vi "XY Plot Commands.vi"(1 "X,Y Log":i32[](array[numeric])=[1, 0], 3 "input string":string="Display 'y_#wave#' vs 'x_#wave#'\nAppendToGraph 'y_#wave#' vs 'x_#wave#'\nLabel bottom \"#labelX#\"\nLabel left \"#labelY#\"\nModifyGraph rgb('y_#wave#')=(#r#,#g#,#b#)\n\\\\s('y_#wave#') #label#\nModifyGraph mirror=1\nModifyGraph width=216\nModifyGraph height={Aspect,0.6}\nModifyGraph Log(bottom)=#bottomlog#\nModifyGraph Log(left)=#leftlog#", 4 "Plot labels":string[](array[string])=["SR810 cables", "SR810 cables + 1&2", "detector", "cables", "cables + 1&2", "cables + 2&3", "cables + 3&4"], 5 "X,Y Labels":string[](array[string])=["frequency (Hz)", "V\\Brms\\M (V)"], 6 "wavenames":string[](array[string])=["Sum.000003SR810cables", "Sum.000003SR810cables + 1&2", "Sum.000003detector", "Sum.000003cables", "Sum.000003cables+ 1&2", "Sum.000003cables+ 2&3", "Sum.000003cables+ 3&4"]) -> (0 "result string":string="Display 'y_Sum.000003SR810cables' vs 'x_Sum.000003SR810cables'\nAppendToGraph 'y_Sum.000003SR810cables + 1&2' vs 'x_Sum.000003SR810cables + 1&2'\nAppendToGraph 'y_Sum.000003detector' vs 'x_Sum.000003detector'\nAppendToGraph 'y_Sum.000003cables' vs 'x_Sum.000003cables'\nAppendToGraph 'y_Sum.000003cables+ 1&2' vs 'x_Sum.000003cables+ 1&2'\nAppendToGraph 'y_Sum.000003cables+ 2&3' vs 'x_Sum.000003cables+ 2&3'\nAppendToGraph 'y_Sum.000003cables+ 3&4' vs 'x_Sum.000003cables+ 3&4'\nLabel bottom \"frequency (Hz)\"\nLabel left \"V\\Brms\\M (V)\"\nModifyGraph rgb('y_Sum.000003SR810cables')=(65280,0,0)\nModifyGraph rgb('y_Sum.000003SR810cables + 1&2')=(65280,50688,0)\nModifyGraph rgb('y_Sum.000003detector')=(29696,65280,0)\nModifyGraph rgb('y_Sum.000003cables')=(0,65280,20992)\nModifyGraph rgb('y_Sum.000003cables+ 1&2')=(0,60928,65280)\nModifyGraph rgb('y_Sum.000003cables+ 2&3')=(0,10240,65280)\nModifyGraph rgb('y_Sum.000003cables+ 3&4')=(40448,0,65280)\nLegend/C/N=text0/J \"\\\\s('y_Sum.000003SR810cables') SR810 cables\\r\\\\s('y_Sum.000003SR810cables + 1&2') SR810 cables + 1&2\\r\\\\s('y_Sum.000003detector') detector\\r\\\\s('y_Sum.000003cables') cables\\r\\\\s('y_Sum.000003cables+ 1&2') cables + 1&2\\r\\\\s('y_Sum.000003cables+ 2&3') cables + 2&3\\r\\\\s('y_Sum.000003cables+ 3&4') cables + 3&4\"\nModifyGraph mirror=1\nModifyGraph width=216\nModifyGraph height={Aspect,0.6}\n\n\n")   [LabVIEW 2016, in "LVtoITX.lvclass"]
uses:
  LVtoITX.lvclass
  <userlib>/LevyLab/Graph Utilities/graph_utilities.lvclass
panel:
  # "Legend/C/N=text0/J \"\\\\s('y_test.000011Plot9') Plot 9\\r\\\\s('y_test.000011Plot8') Plot 8\""
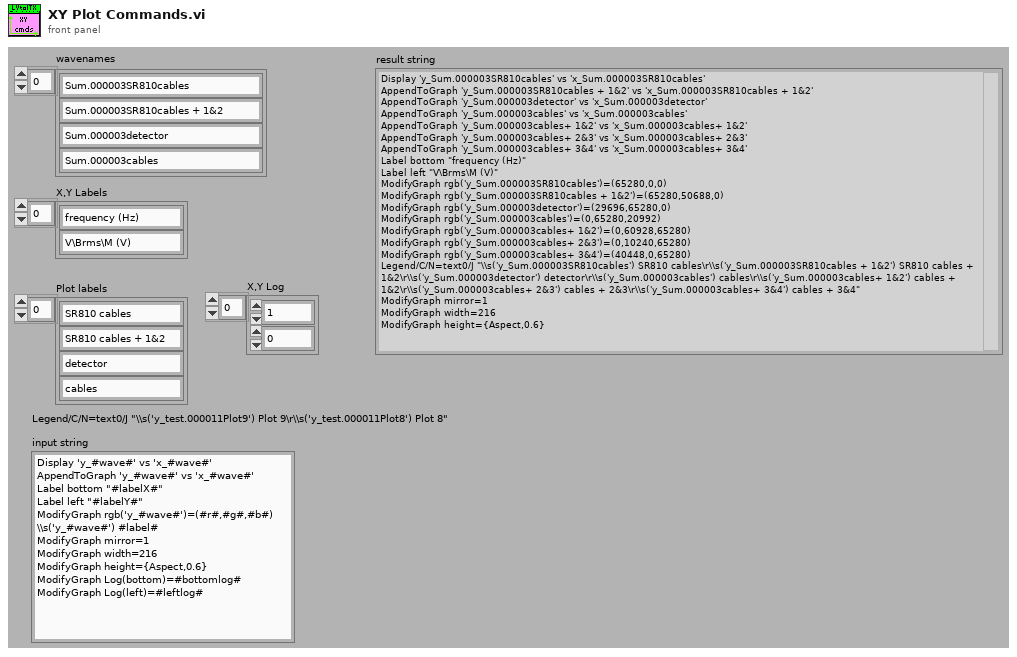
[diagram p1: front panel]
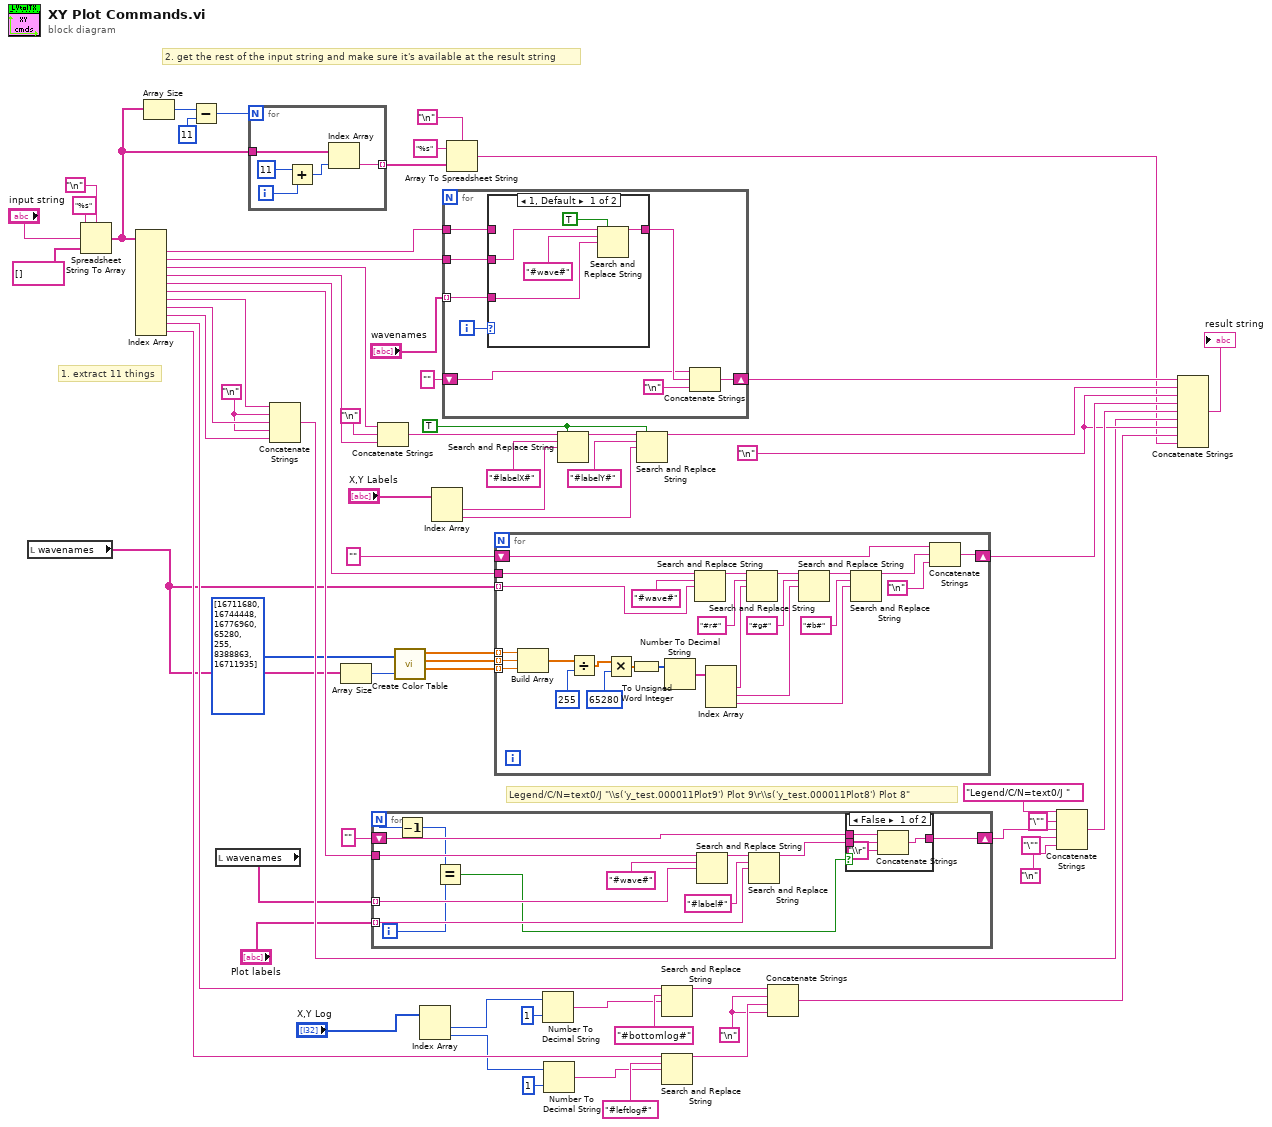
[diagram p0: block diagram]
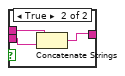
[diagram p2: hidden frame]
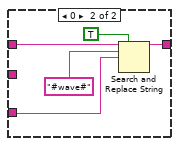
[diagram p3: hidden frame]
diagram:
  w25 = "\n"
  w34 = "\n"
  w33 = "\n"
  w55 = TRUE ("replace all? (F)")
  # "2. get the rest of the input string and make sure it's available at the result string"
  # "1. extract 11 things"
  # "Legend/C/N=text0/J \"\\\\s('y_test.000011Plot9') Plot 9\\r\\\\s('y_test.000011Plot8') Plot 8\""
  n1 = local read "wavenames"() -> (w1:string[])
  n2 = Spreadsheet String To Array(delimiter (Tab)="\n", format string="%s", spreadsheet string="input string", array type (2D Dbl)=string[] []) -> (array=w11:string[])
  n3 = Index Array(array=w11) -> (element #1=w63:string, element #2=w62:string, element #3=w47:string, element #4=w48:string, element #5=w49:string, element #6=w45:string, element #7=w44:string, element #8=w43:string, element #9=w35:string, element #10=w23:string, element #11=w22:string)  [unwired: 11 in]
  n4 = Array Size(array=w11) -> (size(s)=w14:i32)
  n5 = Subtract(x=w14, y=11 ("x")) -> (x-y=w12:i32)
  n6 = local read "wavenames"() -> (w29:string[])
  n7 = for {
    N: w12 -> [_]
    tunnel: w11 -> [w72]
    tunnel: [w71] -> w10 mode=indexing
    i -> [w74]
    n8 = Add(x=11, y=w74) -> (x+y=w75:i32)
    n9 = Index Array(array=w72, index=w75) -> (element=w71:string)
  }
  n10 = Concatenate Strings(w44, w34, w43, w34, w35) -> (w32:string)
  n11 = Array Size(array=w1) -> (size(s)=w6:i32)
  n12 = for {
    N -> [w79]
    shift-right: [w80] -> w38
    shift-left: "" -> [w87]
    tunnel: "Plot labels" -> [w81] mode=indexing
    tunnel: w45 -> [w84]
    tunnel: w29 -> [w83] mode=indexing
    i -> [w77]
    n13 = Decrement(x=w79) -> (x-1=w78:i32)
    n14 = Equal?(x=w78, y=w77) -> (x = y?=w76:bool)
    n15 = Search and Replace String(input string=w84, search string="#wave#", replace string=w83) -> (result string=w88:string)  [unwired: 1 in, 7 out]
    n16 = Search and Replace String(input string=w88, search string="#label#", replace string=w81) -> (result string=w82:string)  [unwired: 1 in, 7 out]
    n17 = case shown="False" w76 {
      tunnel: w87 -> [w92 w94]
      tunnel: w82 -> [w91 w93]
      tunnel: [w90 w95] -> w80
      frame False {
        n18 = Concatenate Strings(w92, w91, "\\r" ("string")) -> (w90:string)
      }
      frame True {
        n19 = Concatenate Strings(w94, w93) -> (w95:string)
      }
    }
  }
  n20 = Concatenate Strings(w47, "\n", w48) -> (w60:string)
  n21 = call <userlib>:"Create Color Table.vi"("Colors []"=u32[] [16711680, 16744448, 16776960, 65280, 255, 8388863, 16711935], "Size (256)"=w6) -> ("R []"=w5:dbl[], "G []"=w4:dbl[], "B []"=w3:dbl[])  [unwired: 1 out]
  n22 = Index Array(array="X,Y Log") -> (element #1=w16:i32, element #2=w15:i32)  [unwired: 2 in]
  n23 = Index Array(array="X,Y Labels") -> (element #1=w51:string, element #2=w50:string)  [unwired: 2 in]
  n24 = for {
    tunnel: "wavenames" -> [w101] mode=indexing
    tunnel: w63 -> [w103]
    tunnel: w62 -> [w102]
    shift-right: [w99] -> w67
    shift-left: "" -> [w96]
    i -> [w100]
    n25 = case shown="1, Default" w100 {
      tunnel: w103 -> [_ w111]
      tunnel: w102 -> [w106 _]
      tunnel: w101 -> [w107 w112]
      tunnel: [w105 w110] -> w98
      frame 1, Default {
        n26 = Search and Replace String(replace all?=TRUE ("replace all? (F)"), input string=w106, search string="#wave#", replace string=w107) -> (result string=w105:string)  [unwired: 1 in, 6 out]
      }
      frame 0 {
        n27 = Search and Replace String(replace all?=TRUE ("replace all? (F)"), input string=w111, search string="#wave#", replace string=w112) -> (result string=w110:string)  [unwired: 1 in, 6 out]
      }
    }
    n28 = Concatenate Strings(w96, w98, "\n") -> (w99:string)
  }
  n29 = Array To Spreadsheet String(delimiter (Tab)="\n", array=w10, 3:"%s" ("format string")) -> (spreadsheet string=w7:string)
  n30 = for {
    tunnel: w49 -> [w133]
    tunnel: w1 -> [w118] mode=indexing
    shift-right: [w130] -> w53
    shift-left: "" -> [w129]
    tunnel: w5 -> [w116] mode=indexing
    tunnel: w4 -> [w115] mode=indexing
    tunnel: w3 -> [w114] mode=indexing
    n31 = Build Array(w116, w115, w114) -> (w117:dbl[])
    n32 = Divide(x=w117, y=255) -> (x/y=w136:dbl[])
    n33 = Multiply(x=w136, y=65280) -> (x*y=w137:dbl[])
    n34 = To Unsigned Word Integer(number=w137) -> (unsigned 16bit integer=w135:u16[])
    n35 = Number To Decimal String(number=w135) -> (decimal integer string=w123:string[])  [unwired: 1 out]
    n36 = Search and Replace String(input string=w133, search string="#wave#", replace string=w118) -> (result string=w134:string)  [unwired: 1 in, 7 out]
    n37 = Index Array(array=w123) -> (element #1=w122:string, element #2=w121:string, element #3=w120:string)  [unwired: 3 in]
    n38 = Search and Replace String(input string=w134, search string="#r#", replace string=w122) -> (result string=w132:string)  [unwired: 1 in, 7 out]
    n39 = Search and Replace String(input string=w132, search string="#g#", replace string=w121) -> (result string=w131:string)  [unwired: 1 in, 7 out]
    n40 = Search and Replace String(input string=w131, search string="#b#", replace string=w120) -> (result string=w127:string)  [unwired: 1 in, 7 out]
    n41 = Concatenate Strings(w129, w127, "\n") -> (w130:string)
  }
  n42 = Number To Decimal String(number=w16, width (-)=i16 1) -> (decimal integer string=w18:string)
  n43 = Number To Decimal String(number=w15, width (-)=i16 1) -> (decimal integer string=w19:string)
  n44 = Search and Replace String(replace all?=w55, input string=w60, search string="#labelX#", replace string=w51) -> (result string=w58:string)  [unwired: 1 in, 6 out]
  n45 = Search and Replace String(replace all?=w55, input string=w58, search string="#labelY#", replace string=w50) -> (result string=w46:string)  [unwired: 1 in, 6 out]
  n46 = Search and Replace String(input string=w23, search string="#bottomlog#", replace string=w18) -> (result string=w27:string)  [unwired: 1 in, 7 out]
  n47 = Search and Replace String(input string=w22, search string="#leftlog#", replace string=w19) -> (result string=w26:string)  [unwired: 1 in, 7 out]
  n48 = Concatenate Strings(w27, w25, w26, w25) -> (w24:string)
  n49 = Concatenate Strings("Legend/C/N=text0/J ", "\"" ("string"), w38, "\"" ("string"), "\n") -> (w40:string)
  n50 = Concatenate Strings(w67, w46, w33, w53, w40, w32, w33, w24, w7) -> (→"result string":string)
